vi "Position Of Center.vi"(7 "VI reference":refnum<vi>, 8 "error in":errorcluster, 11 "Editor Position in":refnum<class "Editor Position.lvclass">) -> (0 "error out":errorcluster, 3 "Editor Position out":refnum<class "Editor Position.lvclass">)   [LabVIEW 2021, in "Editor Position.lvclass"]
uses:
  Editor Position.lvclass
  Editor Position.lvclass/Editor Position.ctl
  4ddca372-28ce-455b-b98e-e0deda970e19.vi
  <vilib>/LabVIEW Icon API/lv_icon/lv_icon.lvlib
  <vilib>/Utility/miscctls.llb/LVRectTypeDef.ctl
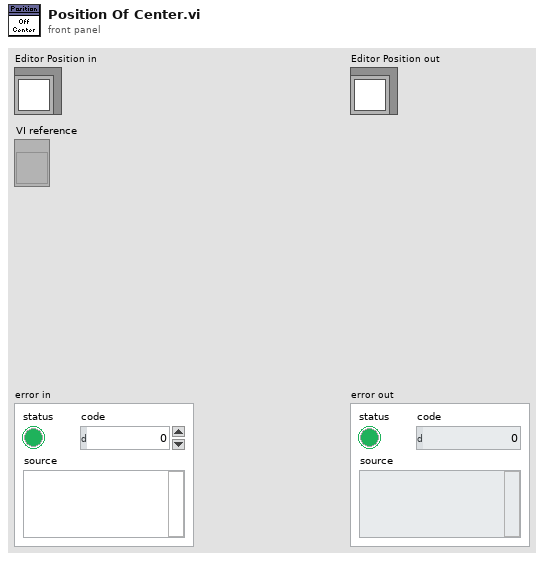
[diagram p1: front panel]
types:
  T1 = typedef "LVRectTypeDef.ctl" = cluster{"Left":i16, "Top":i16, "Right":i16, "Bottom":i16}
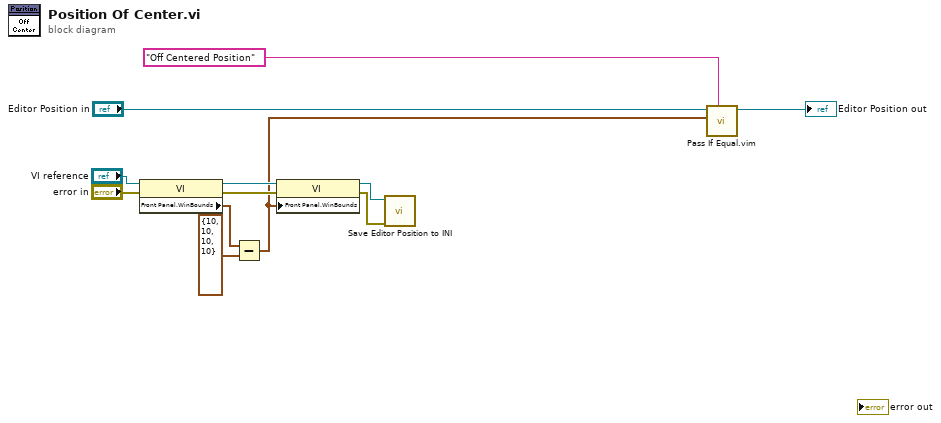
[diagram p0: block diagram]
diagram:
  n1 = property class="VI"(reference="VI reference", error in="error in") -> (reference out=w7:refnum<vi>, error out=w12:errorcluster, "Front Panel.WinBounds"=w6:T1)
  n2 = Subtract(x=w6, y=T1 {"Left"=10, "Top"=10, "Right"=10, "Bottom"=10}) -> (x-y=w2:T1)
  n3 = property class="VI"(reference=w7, error in=w12, "Front Panel.WinBounds"=w2) -> (reference out=w1:refnum<vi>, error out=w11:errorcluster)
  n4 = call <resource>:"Save Editor Position to INI.vi"("error in"=w11, 11:w1) -> ()  [unwired: 9 in, 1 out]
  n5 = call "Pass If Equal.vim"("Description"="Off Centered Position", "Expected"=w2, "LUnit Test Case In"="Editor Position in") -> ("LUnit Test Case Out"=→"Editor Position out":refnum<class "Editor Position.lvclass">)  [unwired: 7 in, 1 out]
